vi "Canonicalize Path.vi"(6 "timeout (ms)":i32=30000, 8 "error in":errorcluster, 10 "path":string, 11 "session in":refnum<class "Session.lvclass">) -> (0 "error out":errorcluster, 2 "canonicalized path":string, 3 "session out":refnum<class "Session.lvclass">)   [LabVIEW 2020, in "NI_SFTP.lvlib"]
doc: "Transform <b>path</b> into its canonical form. The returned path is absolute."
uses:
  <vilib>/net/SFTP/NI_SFTP.lvlib
  <vilib>/net/SFTP/Session/Session.lvclass
  <vilib>/net/SFTP/API/Support/Command/SSH_FXP_REALPATH/SSH_FXP_REALPATH.lvclass
  <vilib>/Utility/Deadline/NI_Deadline.lvlib
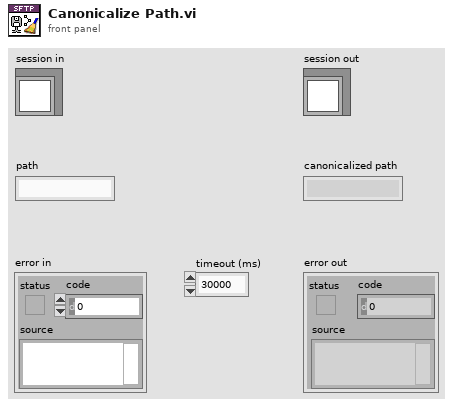
[diagram p1: front panel]
types:
  T1 = typedef "NI_Deadline.lvlib/Deadline.ctl" = cluster{"mode":T2, "deadline (ms)":u32}
  T2 = typedef "NI_Deadline.lvlib/Mode.ctl" = enum16{"Relative", "Use deadline", "Wait forever", "Nonblocking", "N/A"}
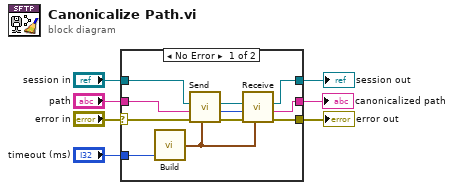
[diagram p0: block diagram]
diagram:
  n1 = case shown="No Error" "error in" {
    selector: "error in" -> [w18 w20]
    tunnel: [w14 w20] -> w6
    tunnel: [w10 w19] -> w4
    tunnel: "session in" -> [w9 w19]
    tunnel: "path" -> [w8 _]
    tunnel: "timeout (ms)" -> [w17 _]
    tunnel: [w11 _] -> w1
    frame No Error {
      n2 = call <vilib>:"Build.vi"("timeout (ms)"=w17) -> ("Deadline out"=w13:T1)  [unwired: 2 in]
      n3 = call <vilib>:"Send.vi"("Timeout"=w13, "error in (no error)"=w18, "path"=w8, "session in"=w9) -> ("error out"=w15:errorcluster, "request id"=w12:u32, "session out"=w16:refnum<class "Session.lvclass">)  [unwired: 4 in, 1 out]
      n4 = call <vilib>:"Receive.vi"("deadline"=w13, "error in (no error)"=w15, "request id"=w12, "session in"=w16) -> ("error out"=w14:errorcluster, "path"=w11:string, "session out"=w10:refnum<class "Session.lvclass">)  [unwired: 4 in, 1 out]
    }
    frame Error {
    }
  }
  "error out" <- w6
  "session out" <- w4
  "canonicalized path" <- w1
